vi "icolor1.vi"(4 "error in (no error)":errorcluster, 7 "Bool Refnum":refnum<vi>) -> ()   [LabVIEW 2010]
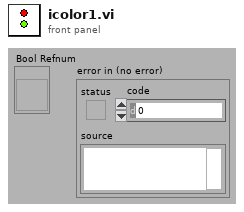
[diagram p1: front panel]
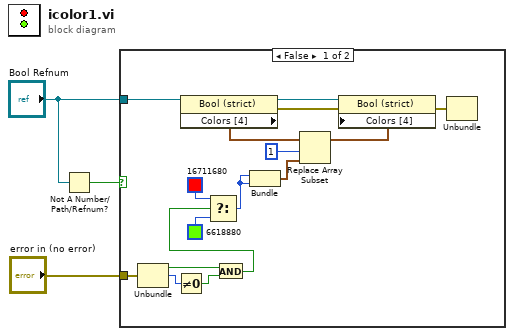
[diagram p0: block diagram]
diagram:
  n1 = Not A Number/Path/Refnum?(number/path/refnum="Bool Refnum") -> (NaN/Path/Refnum?=w1:bool)
  n2 = case shown="False" w1 {
    tunnel: "error in (no error)" -> [w11 _]
    tunnel: "Bool Refnum" -> [w4 _]
    frame False {
      n3 = Unbundle(w11) -> ("status"=w8:bool, "code"=w10:i32)  [unwired: 1 out]
      n4 = Not Equal To 0?(x=w10) -> (x != 0?=w9:bool)
      n5 = property on="Property Node" class="Bool (strict)"(reference=w4) -> (error out=w6:errorcluster, "Colors [4]"=w16:cluster{u32, u32}[])  [unwired: 1 in, 1 out]
      n6 = And(x=w8, y=w9) -> (x .and. y?=w7:bool)
      n7 = Select(t=u32 16711680 ("Color Box"), s=w7, f=u32 6618880 ("Color Box")) -> (s? t:f=w13:u32)
      n8 = Bundle("Color Box"=w13, "Color Box"=w13) -> (w17:cluster{"Color Box":u32, "Color Box":u32})  [unwired: 1 in]
      n9 = Replace Array Subset(array=w16, new element=w17, index=1) -> (w12:cluster{u32, u32}[])
      n10 = property on="Property Node" class="Bool (strict)"(reference=w4, error in=w6, "Colors [4]"=w12) -> (error out=w5:errorcluster)  [unwired: 1 out]
      n11 = Unbundle(w5) -> ()  [unwired: 3 out]
    }
    frame True {
    }
  }
